vi "Run Tests (Test Object Array).vi"(7 "TextTestRunner in":refnum<class "TextTestRunner.lvclass">, 8 "error in (no error)":errorcluster, 10 "Tests":refnum<class>[](array[class])) -> (0 "error out":errorcluster, 1 "test details":string, 2 "successful?":bool)   [LabVIEW 2011, in "VI Tester API.lvlib"]
doc: "Run test classes (TestCase or TestSuites). Tests are test objects -- for example from test object constants on a block diagram."
uses:
  VI Tester API.lvlib
  Classes/TextTestRunner/TextTestRunner.lvclass
  Classes/TestLoader/TestLoader.lvclass
  Classes/TestResult/TestResult.lvclass
panel:
  # "JKI VI Tester for LabVIEW\nhttp://jkisoft.com/vi-tester\nCopyright (C) 2007-2009, JKI <info@jkisoft.com>\nALL RIGHTS RESERVED"
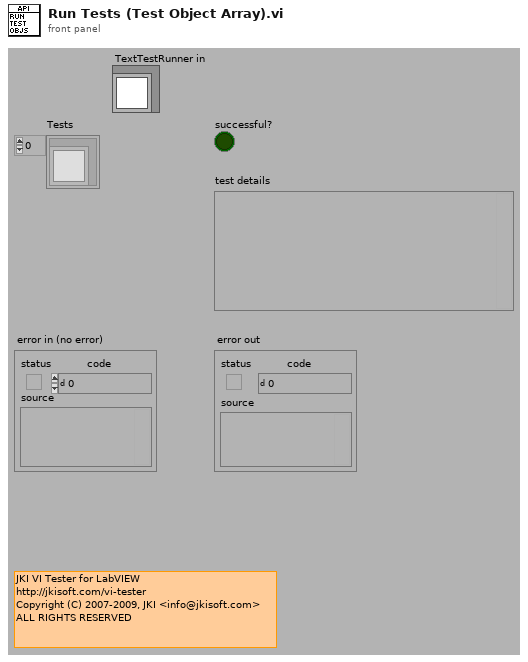
[diagram p1: front panel]
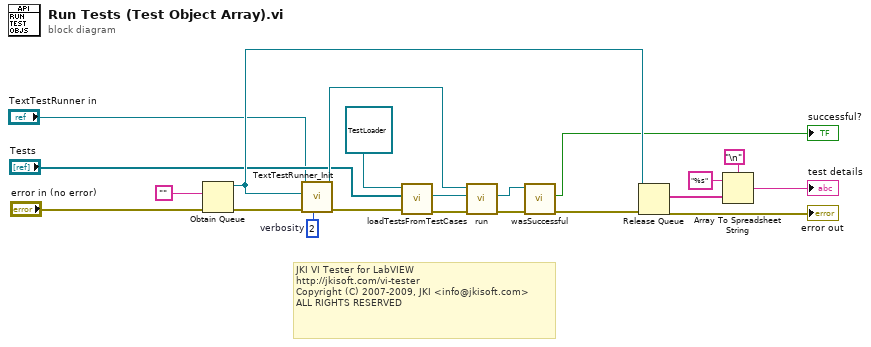
[diagram p0: block diagram]
diagram:
  w8 = u32 2  # verbosity
  # "JKI VI Tester for LabVIEW\nhttp://jkisoft.com/vi-tester\nCopyright (C) 2007-2009, JKI <info@jkisoft.com>\nALL RIGHTS RESERVED"
  n1 = Obtain Queue(element data type="", error in (no error)="error in (no error)") -> (queue out=w16:refnum<queue>, error out=w10:errorcluster)  [unwired: 3 in, 1 out]
  n2 = call "TextTestRunner_Init.vi"("verbosity (1)"=w8, "error in (no error)"=w10, "stream"=w16, "TextTestRunner in"="TextTestRunner in") -> ("error out"=w21:errorcluster, "TextTestRunner out"=w11:refnum<class "TextTestRunner.lvclass">)  [unwired: 6 in]
  n3 = call-dynamic "loadTestsFromTestCases.vi"("error in (no error)"=w21, "Tests"="Tests", "TestLoader in"=refnum<class "TestLoader.lvclass"> refnum ("reference in")) -> ("error out"=w12:errorcluster, "TestSuite"=w7:refnum<class "TestSuite.lvclass">)  [unwired: 6 in, 1 out]
  n4 = call-dynamic "run.vi"("error in (no error)"=w12, "test"=w7, "TextTestRunner in"=w11) -> ("error out"=w14:errorcluster, "TestResult out"=w13:refnum<class "TestResult.lvclass">)  [unwired: 6 in, 1 out]
  n5 = call-dynamic "wasSuccessful.vi"("error in (no error)"=w14, "TestResult in"=w13) -> ("error out"=w4:errorcluster, "successful?"=→"successful?":bool)  [unwired: 7 in, 1 out]
  n6 = Release Queue(queue=w16, error in (no error)=w4) -> (remaining elements=w17:string[], error out=→"error out":errorcluster)  [unwired: 1 in, 1 out]
  n7 = Array To Spreadsheet String(delimiter (Tab)="\n", array=w17, 3:"%s" ("format string")) -> (spreadsheet string=→"test details":string)
